vi "Print.vi"(11 "CANopen Message in":refnum<class "CANopen Message.lvclass">) -> (2 "Message":string, 3 "CANopen Message out":refnum<class "CANopen Message.lvclass">)   [LabVIEW 2024, in "CANopen Master.lvlib" / "CANopen Message.lvclass"]
uses:
  CANopen Message.lvclass
  CANopen Message.lvclass/CANopen Message.ctl
  <vilib>/Utility/error.llb/whitespace.ctl
  Timestamp/Timestamp.lvclass
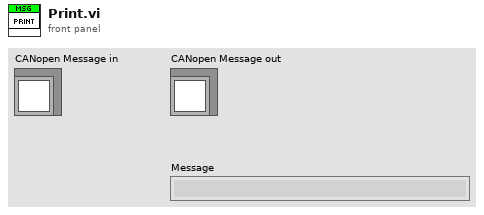
[diagram p1: front panel]
types:
  T1 = typedef "whitespace.ctl" = u16
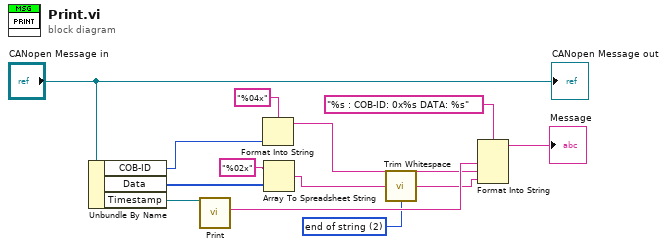
[diagram p0: block diagram]
diagram:
  w1 = T1 2 items=["both", "start of string", "end of string"] ("location (both)")
  n1 = Unbundle By Name("CANopen Message in") -> ("COB-ID"=w9:u32, "Data"=w10:u8[], "Timestamp"=w12:refnum<class "Timestamp.lvclass">)
  n2 = call "Print.vi"("Timestamp in"=w12) -> ("Time Stamp"=w7:string)  [unwired: 9 in, 1 out]
  n3 = Format Into String(format string="%04x", w9) -> (resulting string=w6:string)  [unwired: 2 in, 1 out]
  n4 = Array To Spreadsheet String(array=w10, 3:"%02x" ("format string")) -> (spreadsheet string=w3:string)  [unwired: 1 in]
  n5 = call <vilib>:"Trim Whitespace.vi"("string"=w3, "location (both)"=w1) -> ("trimmed string"=w2:string)
  n6 = Format Into String(format string="%s : COB-ID: 0x%s DATA: %s", w7, w6, w2) -> (resulting string=→"Message":string)  [unwired: 2 in, 1 out]
  "CANopen Message out" <- "CANopen Message in"
